vi "sendFIFO.vi"(8 "error in (no error)":errorcluster, 11 "Mockbus in":refnum<class "Mockbus.lvclass">) -> (0 "error out":errorcluster, 3 "Mockbus out":refnum<class "Mockbus.lvclass">)   [LabVIEW 2015, in "RTMockbus.lvlib" / "Mockbus.lvclass"]
uses:
  Mockbus.lvclass
  Mockbus.lvclass/Mockbus.ctl
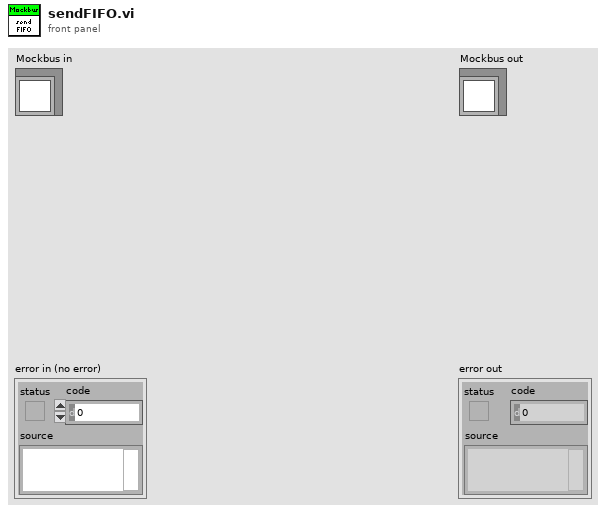
[diagram p1: front panel]
types:
  T1 = typedef "RTModbus.lvlib/Frame.ctl" = cluster{"Data":u8[], "WaitForTrigger":bool, "WaitForRx":u16, "TriggerIRQ":bool, "DelayTicks":u16, "DelayMicroseconds":u16, "DelayMilliseconds":u16}
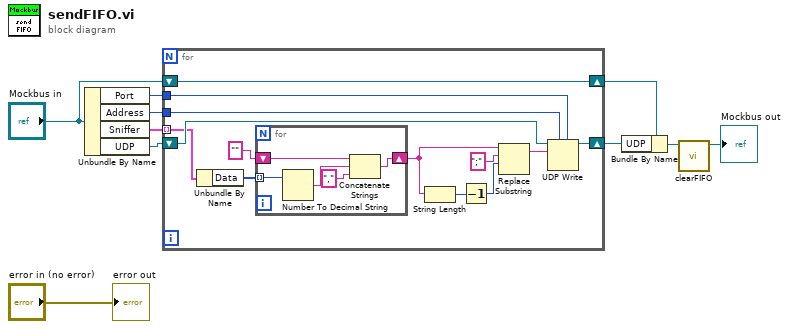
[diagram p0: block diagram]
diagram:
  n1 = Unbundle By Name("Mockbus in") -> ("Port"=w1:u16, "Address"=w2:u32, "Sniffer"=w9:T1[], "UDP"=w8:refnum<k16>)
  n2 = for {
    tunnel: w9 -> [w22] mode=indexing
    shift-right: [w14] -> w3
    shift-left: w8 -> [w23]
    tunnel: w2 -> [w13]
    tunnel: w1 -> [w12]
    shift-right: [w15] -> w5
    shift-left: "Mockbus in" -> [w15]
    n3 = Unbundle By Name(w22) -> ("Data"=w11:u8[])
    n4 = for {
      tunnel: w11 -> [w28] mode=indexing
      shift-right: [w25] -> w19
      shift-left: "" -> [w26]
      n5 = Number To Decimal String(number=w28) -> (decimal integer string=w27:string)  [unwired: 1 in]
      n6 = Concatenate Strings(w26, w27, "," ("string")) -> (w25:string)
    }
    n7 = String Length(string=w19) -> (length=w17:i32)
    n8 = Decrement(x=w17) -> (x-1=w16:i32)
    n9 = Replace Substring(3:w16, 4:";" ("substring (\"\")"), 5:w19) -> (1:w18:string)  [unwired: 1 in, 1 out]
    n10 = UDP Write(address=w13, port or service name=w12, connection ID=w23, data in=w18) -> (3:w14:refnum<k16>)  [unwired: 2 in, 1 out]
  }
  n11 = Bundle By Name(cluster=w5, "UDP"=w3) -> (w4:refnum<class "Mockbus.lvclass">)
  n12 = call "clearFIFO.vi"("Mockbus in"=w4) -> ("Mockbus out"=→"Mockbus out":refnum<class "Mockbus.lvclass">)  [unwired: 9 in, 1 out]
  "error out" <- "error in (no error)"
